vi "DAQ_LED.vi"() -> ()   [LabVIEW 2012]
panel:
  in  "stop":bool
  out "Array":bool[](array[boolean])
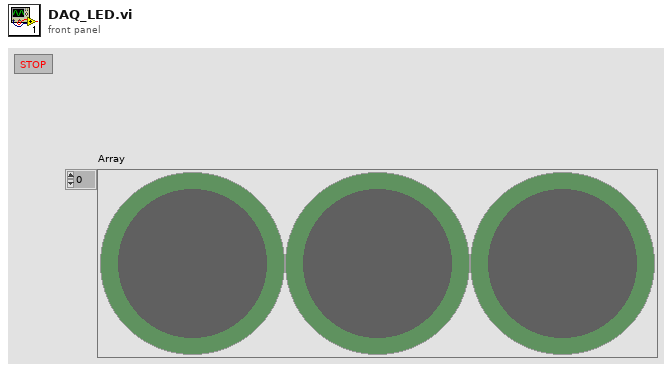
[diagram p1: front panel]
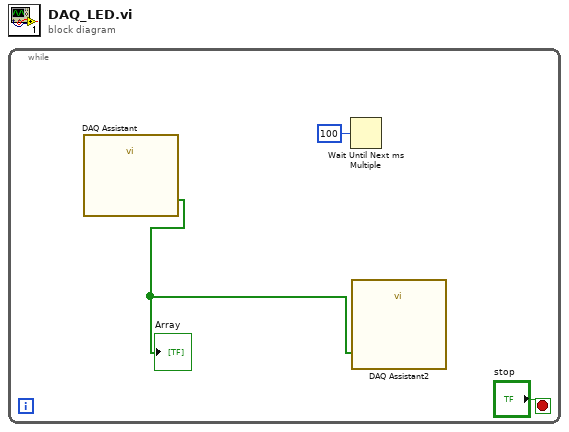
[diagram p0: block diagram]
diagram:
  n1 = while {
    stop <- "stop" stop-if-true
    n2 = call "DAQ Assistant"() -> ("data"=w3:bool[])  [unwired: 17 in, 2 out]
    "Array" <- w3
    n3 = Wait Until Next ms Multiple(millisecond multiple=u32 100) -> ()  [unwired: 1 out]
    n4 = call "DAQ Assistant2"("data"=w3) -> ()  [unwired: 17 in, 2 out]
  }
